vi "Process.vi"(0 "reference in":refnum<class "ACIR_EIS.lvclass">, 5 "error in":errorcluster) -> (14 "reference out":refnum<class "ACIR_EIS.lvclass">, 19 "error out":errorcluster)   [LabVIEW 2023, in "ACIR_EIS.lvclass"]
uses:
  ACIR_EIS.lvclass
  Types/EIS Mode.ctl
  Types/EIS Parameters.ctl
  Logger_class/Logger.lvclass
  <instrlib>/HPS-17000/HPS-17000.lvclass
  <vilib>/HPS-17000/nibatterycycler_grpc_Setpoint.ctl
  <vilib>/HPS-17000/Setpoint Stream Basic Config.ctl
  <vilib>/Utility/NIReport.llb/Report Type.ctl
  <instrlib>/HPS-17000/Internal/Set Energized Multi.vi
  <instrlib>/HPS-17000/Internal/Wait Until Energized Multi.vi
  <instrlib>/HPS-17000/Internal/Read Measurement Multi.vi
  <instrlib>/HPS-17000/Internal/Set Enabled Output Multi.vi
  <instrlib>/HPS-17000/Internal/Start Setpoint Stream Multi.vi
  <instrlib>/HPS-17000/Internal/Stream Setpoints Multi.vi
  <instrlib>/HPS-17000/Internal/Stop Setpoint Stream Multi.vi
  <instrlib>/HPS-17000/Internal/Write Setpoint Multi.vi
  <vilib>/printing/OpenHTMLReport.llb/Open HTML Report in Browser (Refnum).vi
  <vilib>/Utility/NIReport.llb/NI_report.lvclass
  ACIR_EIS.lvclass/ACIR_EIS.ctl
  <vilib>/Utility/SystemLogging/NI_SystemLogging.lvlib
  <vilib>/HPS-17000/NI_BC_client.lvlib
  <userlib>/_OpenG.lib/time/time.llb/openg_time.lvlib
  <vilib>/HPS-17000/Cycler.lvclass
  <vilib>/Utility/NIReport.llb/NI_ReportGenerationCore.lvlib
panel:
  out "Last Command":string
  out "error info":errorcluster
  in  "Save EIS Report":bool
  in  "EIS Tab Control":T1(tab)
  out "EIS Parameters":T3={"EIS Mode"=2, "EIS DC Potential"=650.0, "EIS Start Frequency"=1000.0, "EIS Stop Frequency"=500.0, "EIS Delta Frequency"=100.0, "EIS DC Current"=0.0, "AC Signal (mV/mA RMS)"=20.0, "Cycles at Frequency"=5.0, "EIS AC Step Delay"=1.0} {"EIS Mode" items=["Voltage (PEIS)"=1, "Current (GEIS)"=2]}
  out "EIS Profile":waveform(dbl)[](graph)
  out "Running Status Log":i32(listbox) caption="TEST SERVER LOG"
  out "EIS Step":dbl[][](graph)
  out "EIS Nyquist":cluster{dbl[], dbl[]}(graph)
  out "EIS Phase":cluster{dbl[], dbl[]}(graph)
  out "EIS Magnitude":cluster{dbl[], dbl[]}(graph)
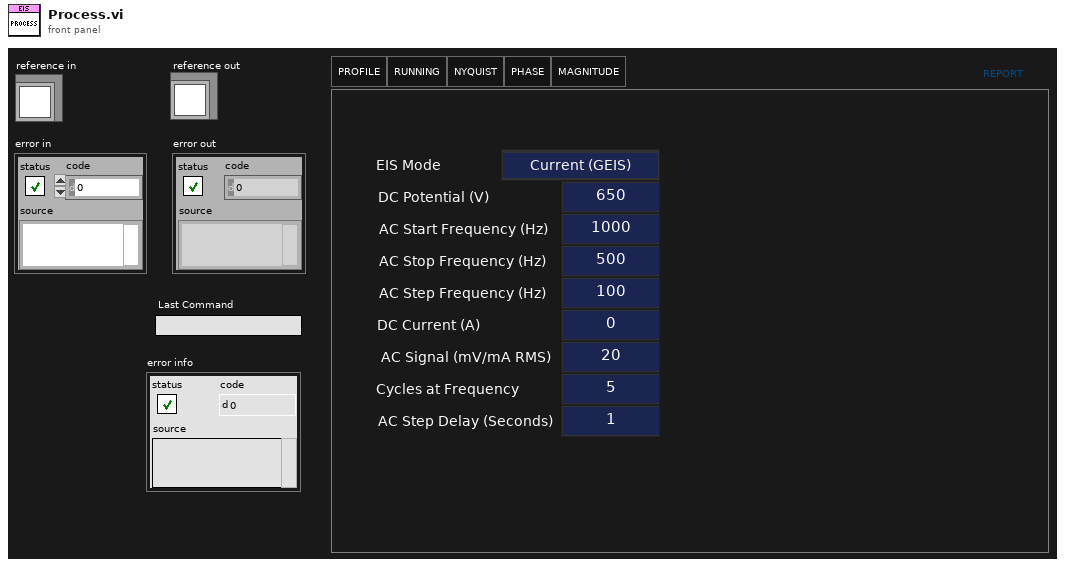
[diagram p1: front panel]
types:
  T1 = enum32{"PARAM", "PROFILE", "RUNNING", "NYQUIST", "PHASE", "MAGNITUDE"}
  T2 = typedef "EIS Mode.ctl" = u16
  T3 = cluster{"EIS Mode":T2, "EIS DC Potential":dbl, "EIS Start Frequency":dbl, "EIS Stop Frequency":dbl, "EIS Delta Frequency":dbl, "EIS DC Current":dbl, "AC Signal (mV/mA RMS)":dbl, "Cycles at Frequency":dbl, "EIS AC Step Delay":dbl}
  T4 = typedef "EIS Parameters.ctl" = cluster{"EIS Mode":T2, "EIS DC Potential":dbl, "EIS Start Frequency":dbl, "EIS Stop Frequency":dbl, "EIS Delta Frequency":dbl, "EIS DC Current":dbl, "AC Signal (mV/mA RMS)":dbl, "Cycles at Frequency":dbl, "EIS AC Step Delay":dbl}
  T5 = cluster{"Core":cluster{"Timeout":i32, "Events":cluster{"EventsToProcess":refnum<event-registration>}, "EventFromProcess":refnum<user-event>, "ProcessSyncQueue":refnum<queue>, "QueueFromProcess":refnum<queue>, "Command":string, "Data":variant}, "EIS Parameters":T4, "Profile Complete Event":refnum<user-event>, "EIS Profile State":enum16{"Idle", "Start", "Run", "Stop"}, "EIS TDMS Path":path, "Logger":refnum<class "Logger.lvclass">, "HPS17K Refs":refnum<class "HPS-17000.lvclass">[], "Voltage Profile":waveform(dbl)[], "Current Profile":waveform(dbl)[], "Next Step Timestamp":i64, "Profile Index":i64, "Frequencies":dbl[]}
  T6 = typedef "Cycler.lvclass/Setpoint Stream Basic Config.ctl" = cluster{"local address":string, "receiver port":u16}
  T7 = typedef "NI_BC_client.lvlib/nibatterycycler_grpc_Setpoint.ctl" = cluster{"voltage":sgl, "current":sgl, "min_power":sgl, "max_power":sgl, "resistance":sgl}
  T8 = enum8{"Enabled", "Disabled", "Disabled and Grayed Out"}
  T9 = typedef "NI_ReportGenerationCore.lvlib/Report Type.ctl" = enum16{"HTML", "Word", "Excel"}
  T10 = enum32{"Invalid", "Standard", "Closed", "Hidden", "Minimized", "Maximized"}
  T11 = cluster{"EventsToProcess":refnum<event-registration>}
  T12 = typedef "NI_BC_client.lvlib/MStream_grpc_CyclerMeasurement.ctl" = cluster{"measured_voltage":sgl, "measured_current":sgl, "setpoint_voltage":sgl, "setpoint_current":sgl, "timestamp":i64}
  T13 = typedef "ACIR_EIS.lvclass/ObjectAttributes.ctl" = cluster{"EIS Parameters":T4, "Logger":refnum<class "Logger.lvclass">, "HPS17K Refs":refnum<class "HPS-17000.lvclass">[]}
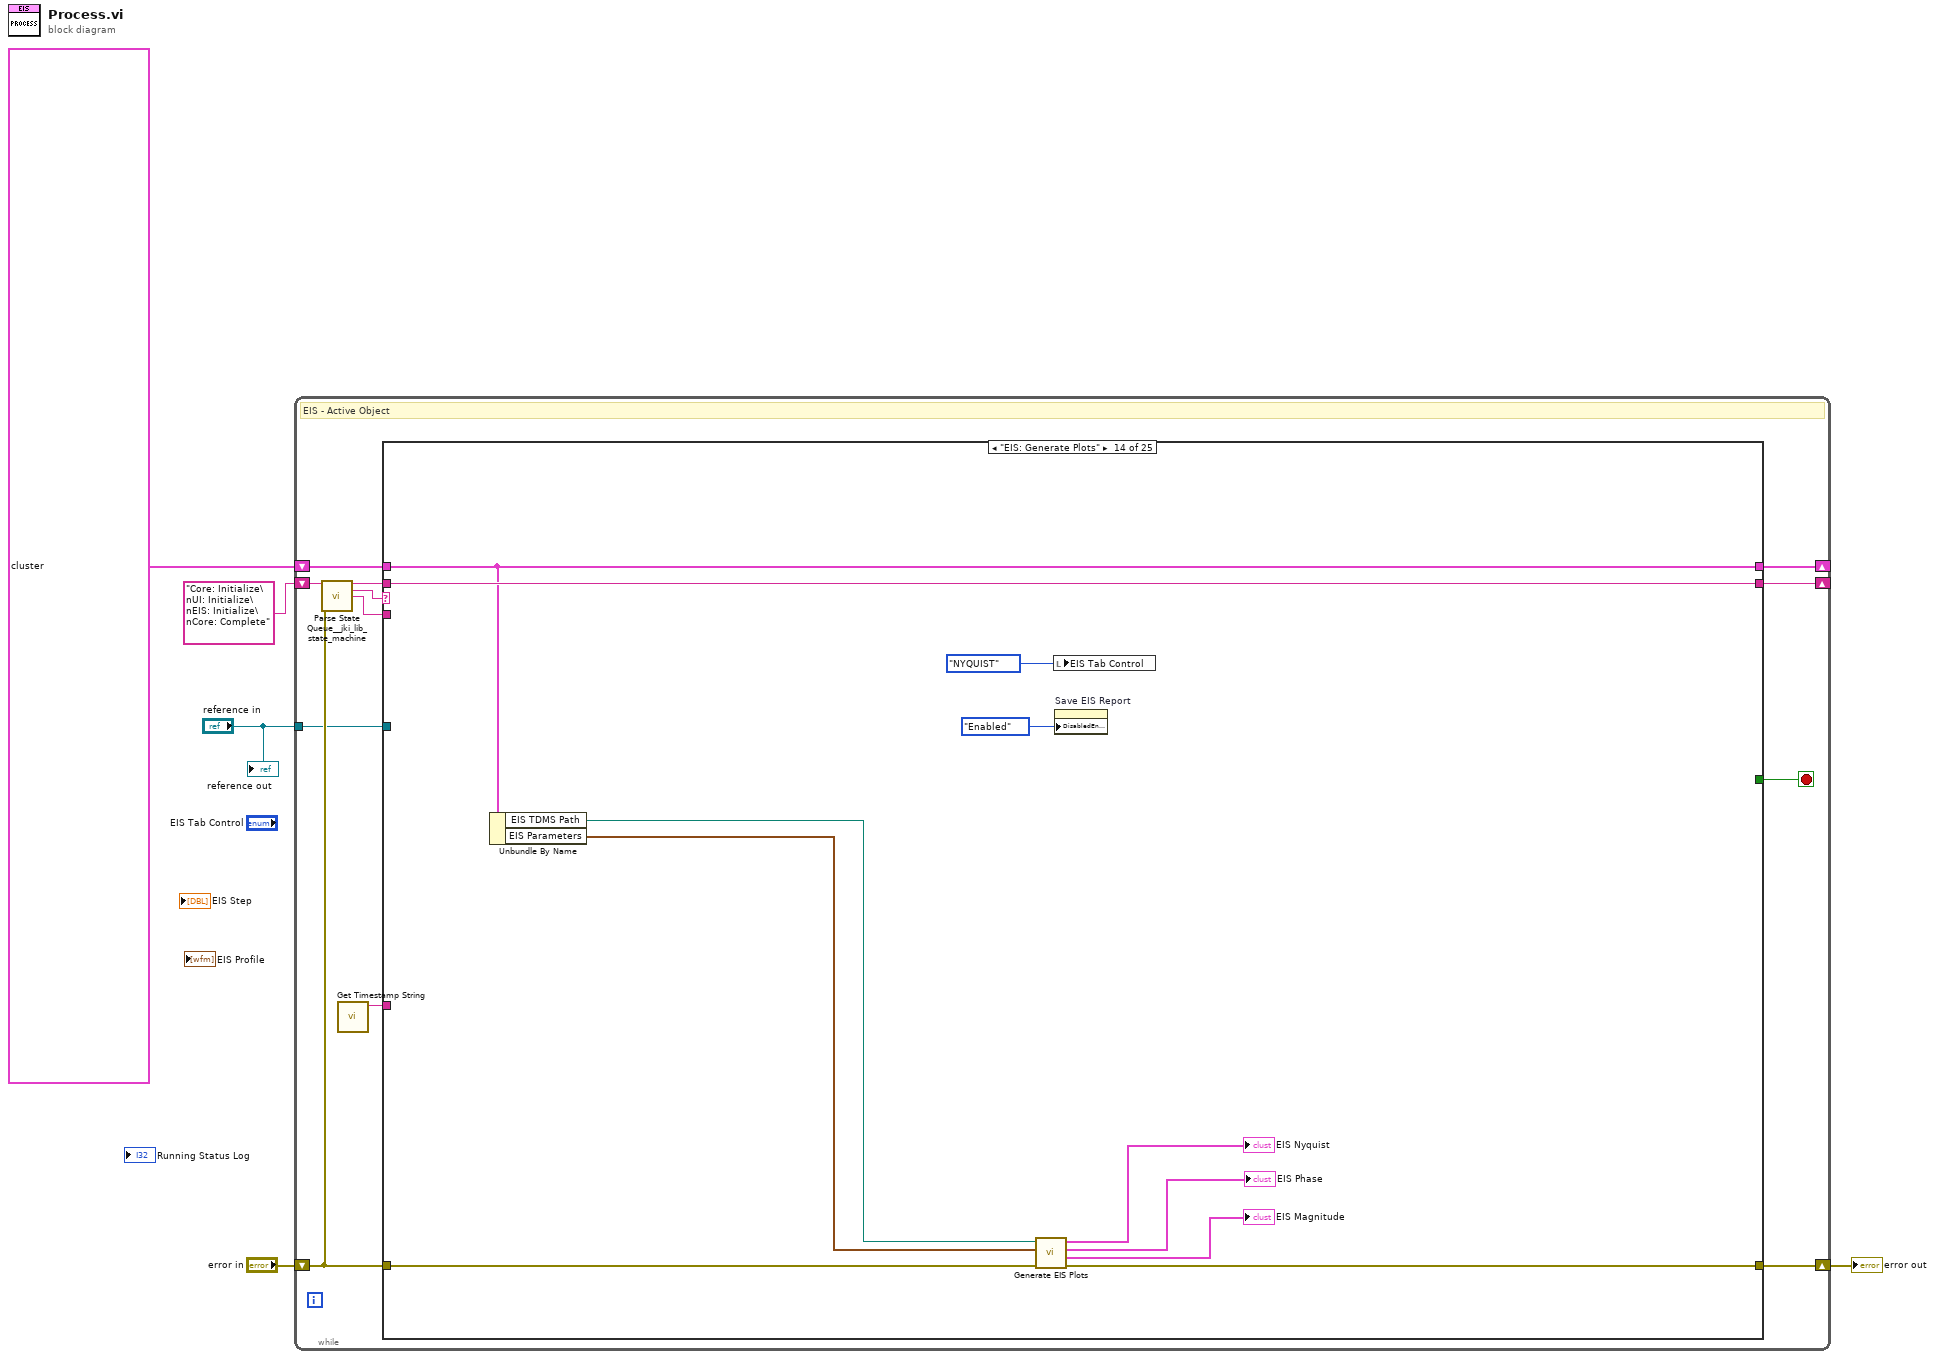
[diagram p0: block diagram]
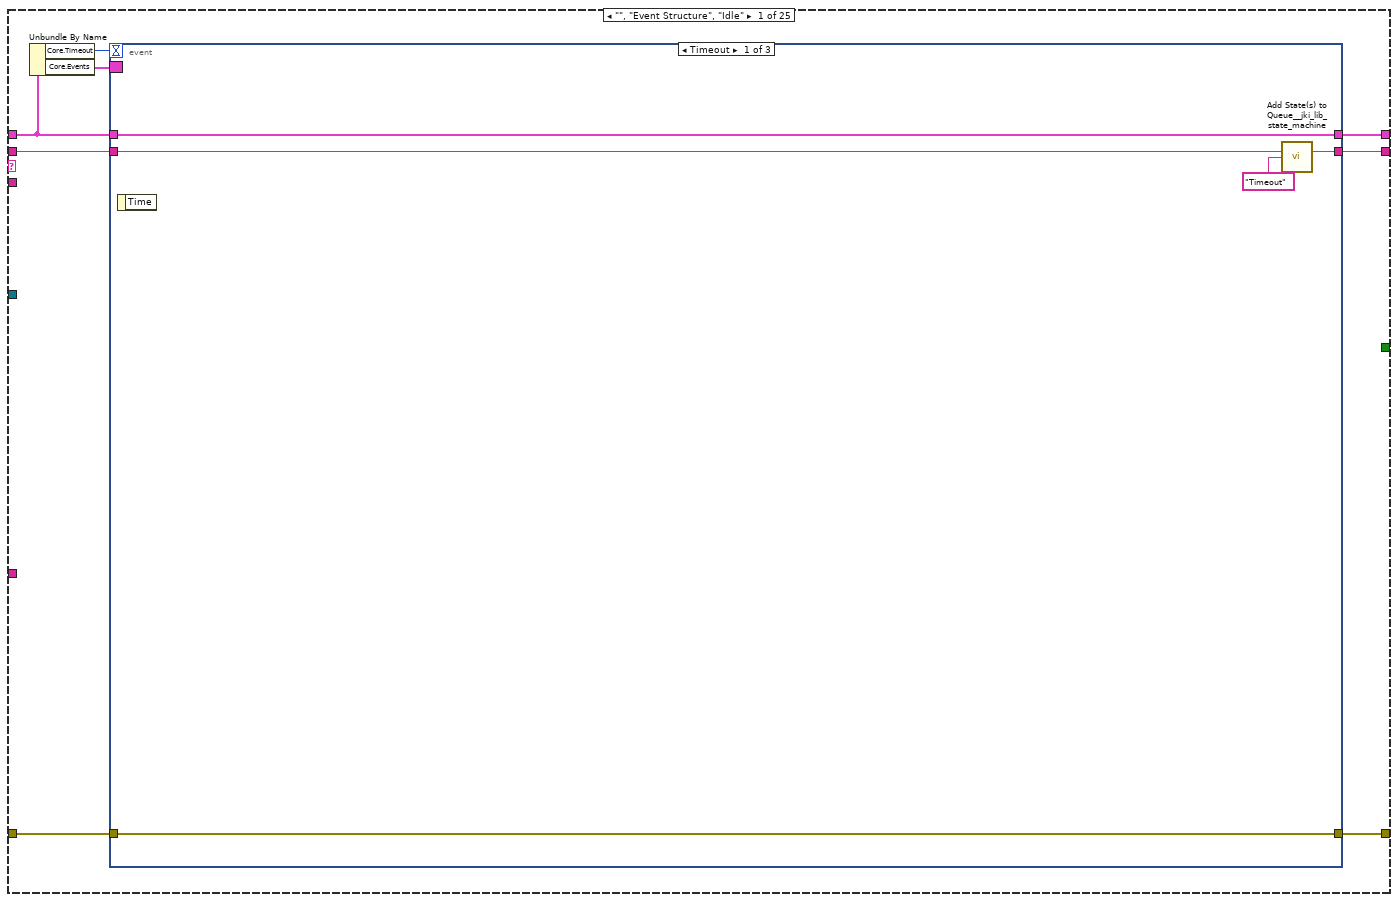
[diagram p2: hidden frame]
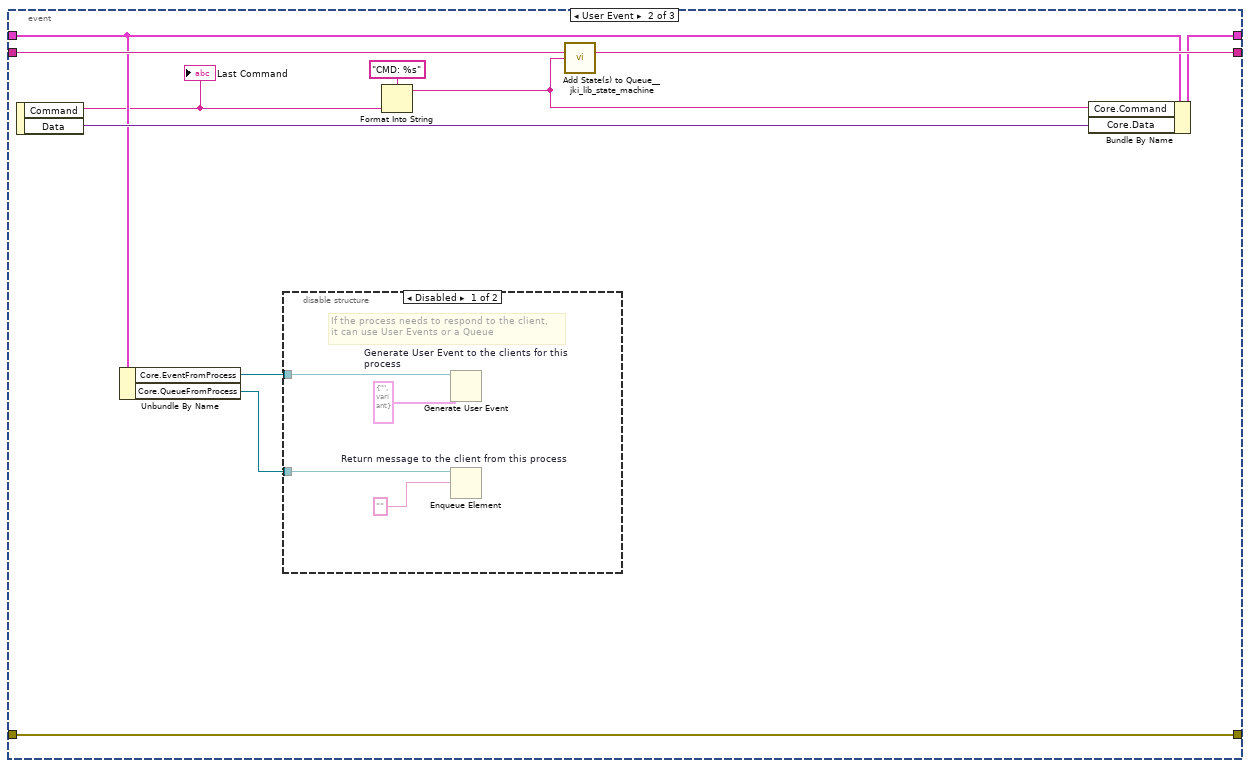
[diagram p3: hidden frame]
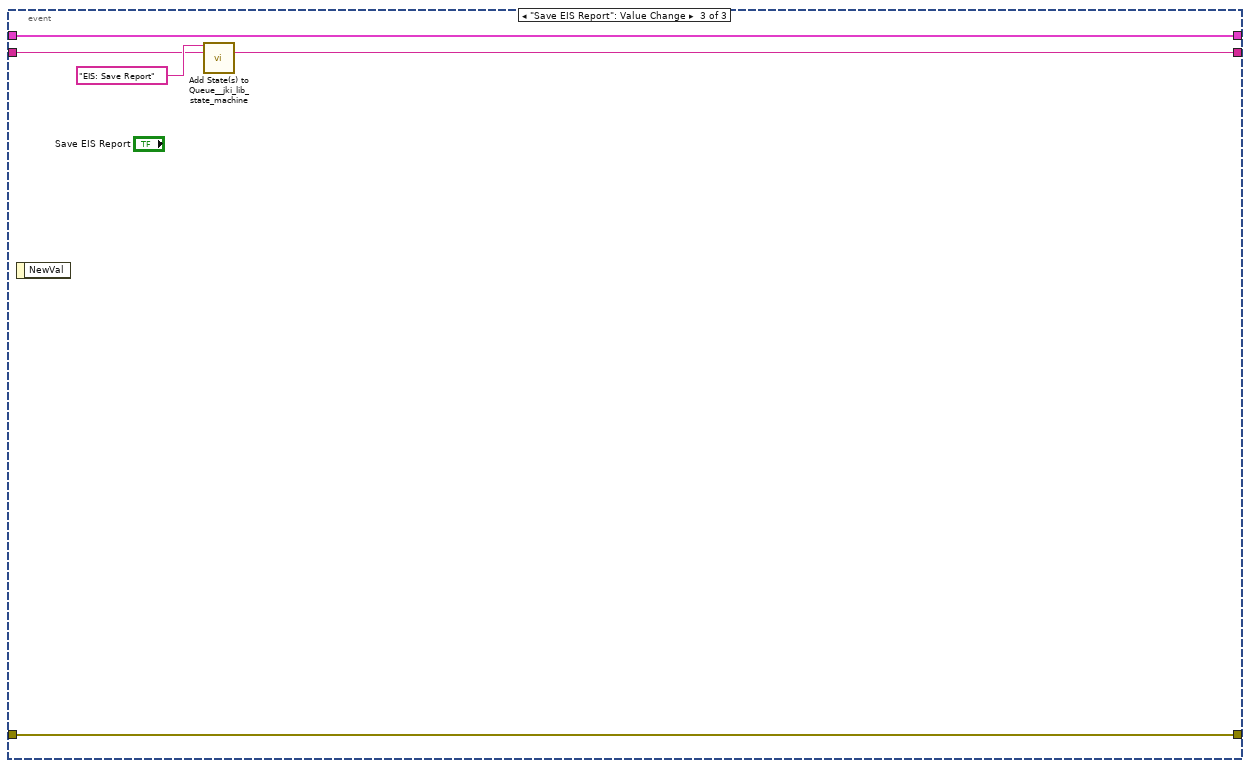
[diagram p5: hidden frame]
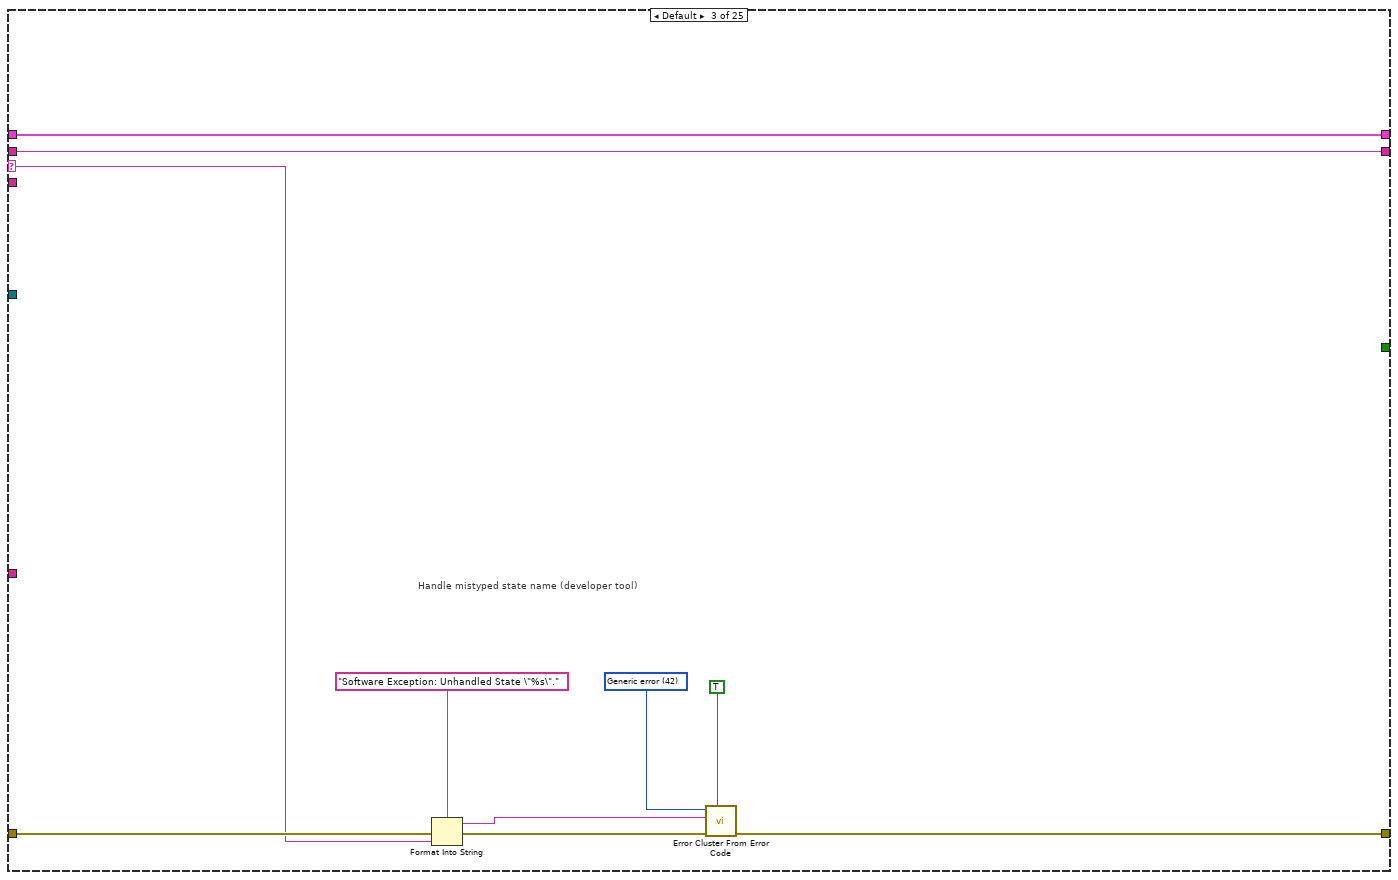
[diagram p7: hidden frame]
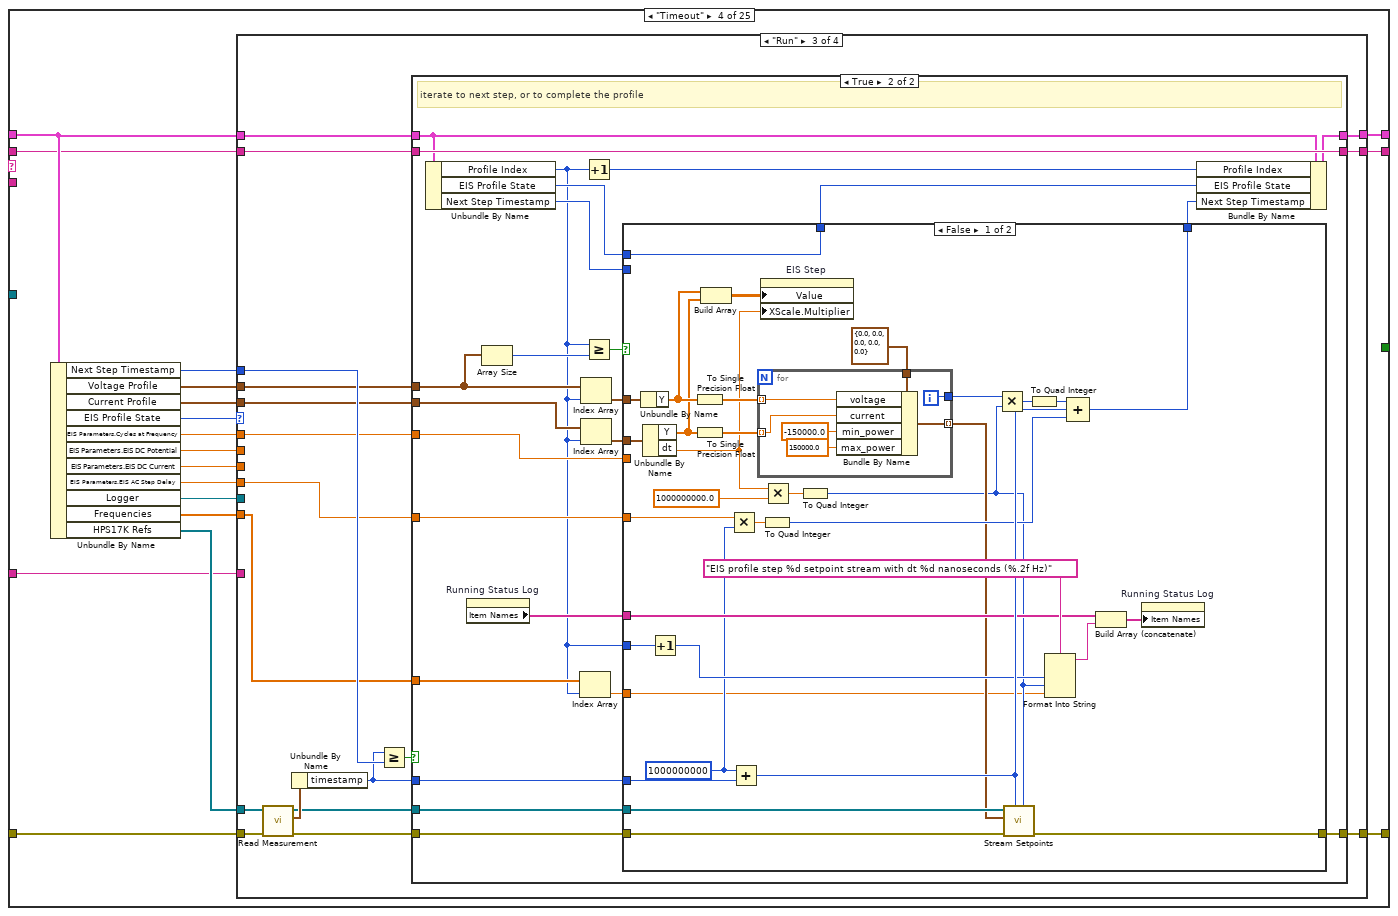
[diagram p8: hidden frame]
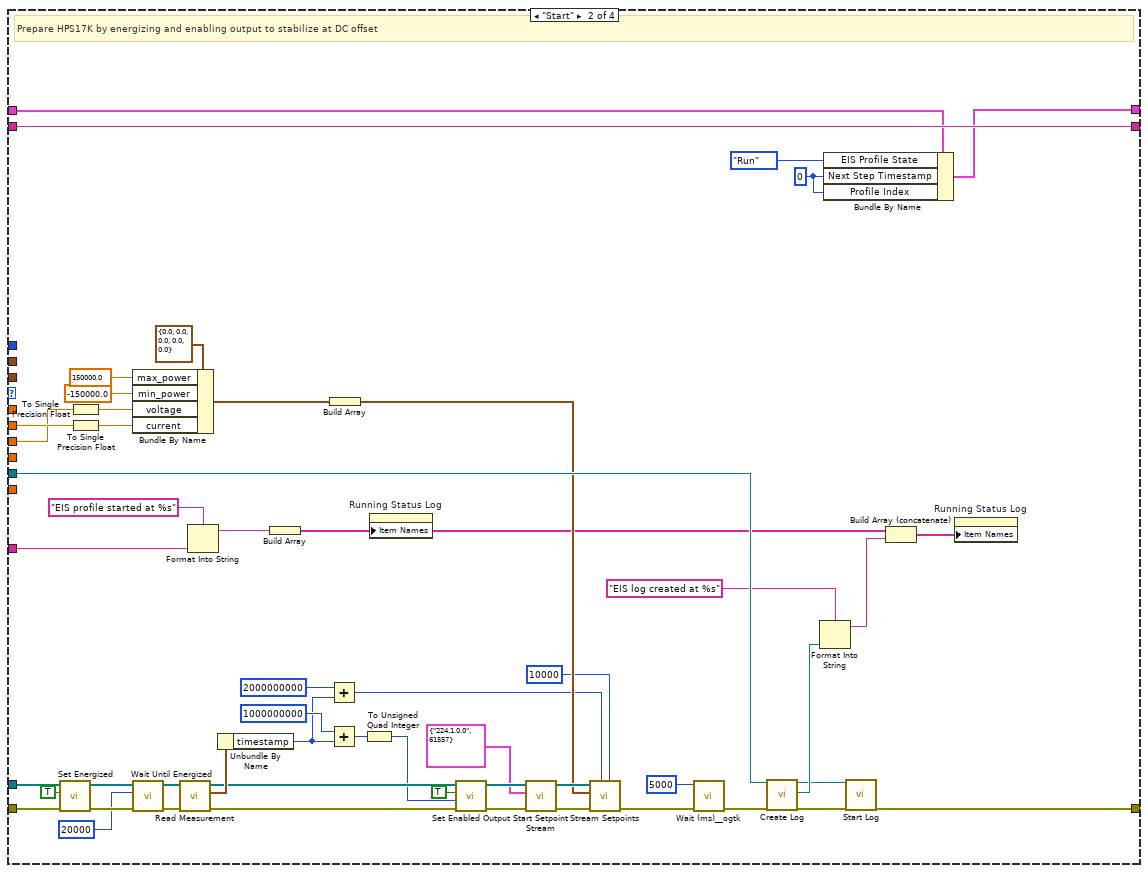
[diagram p10: hidden frame]
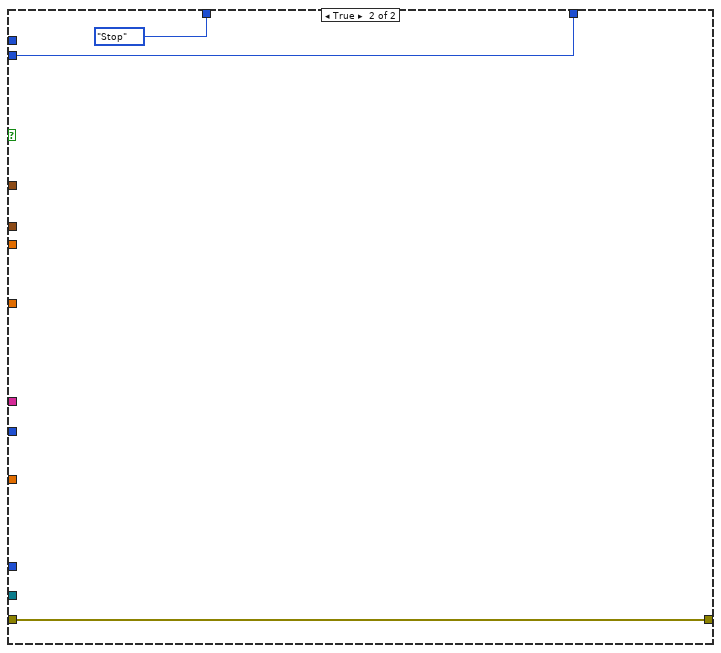
[diagram p12: hidden frame]
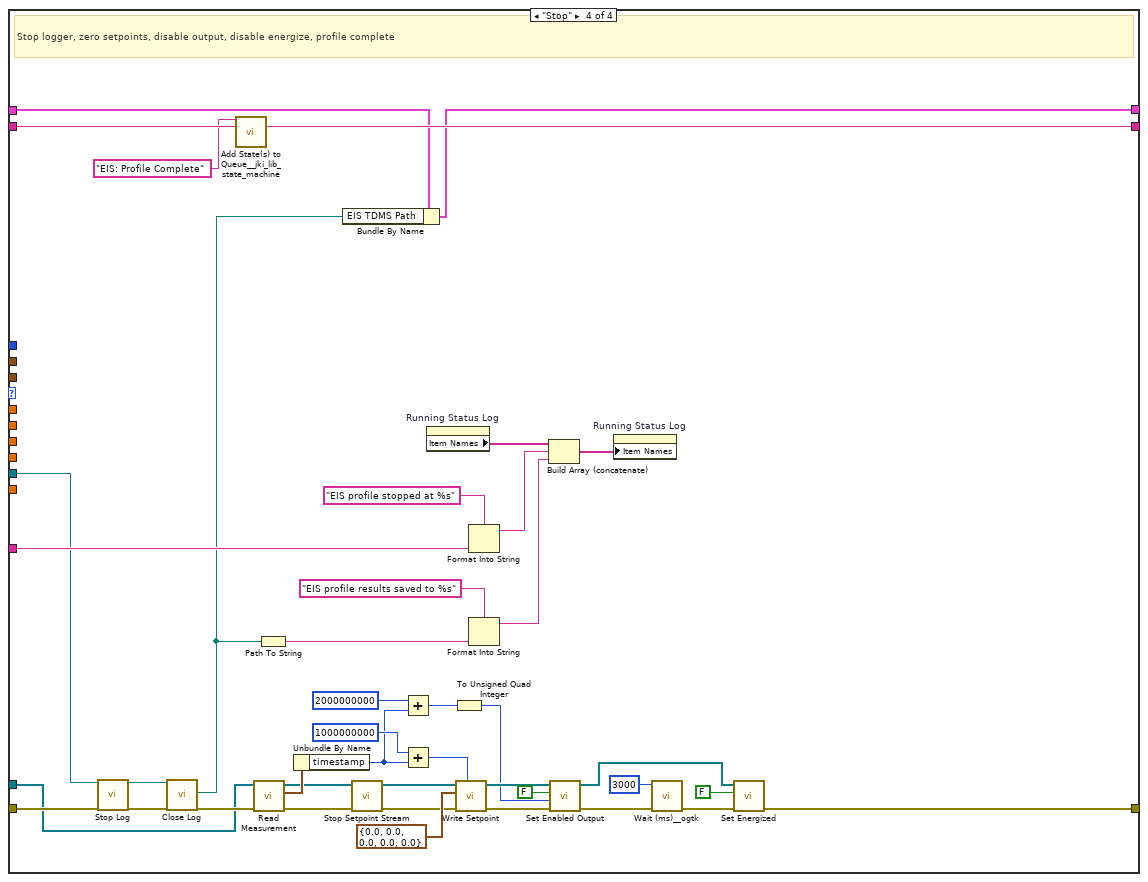
[diagram p13: hidden frame]
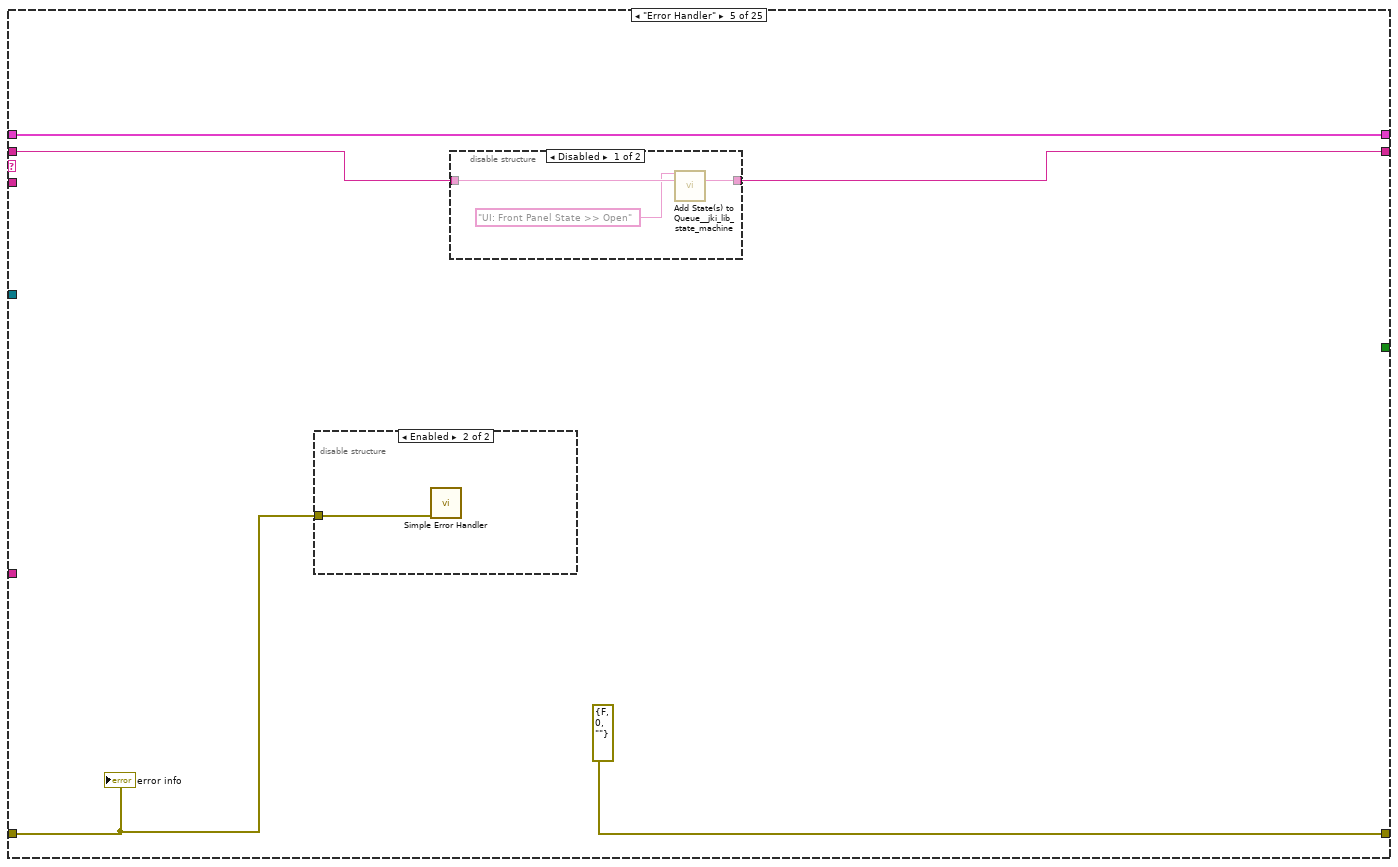
[diagram p14: hidden frame]
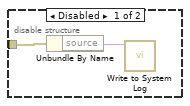
[diagram p16: hidden frame]
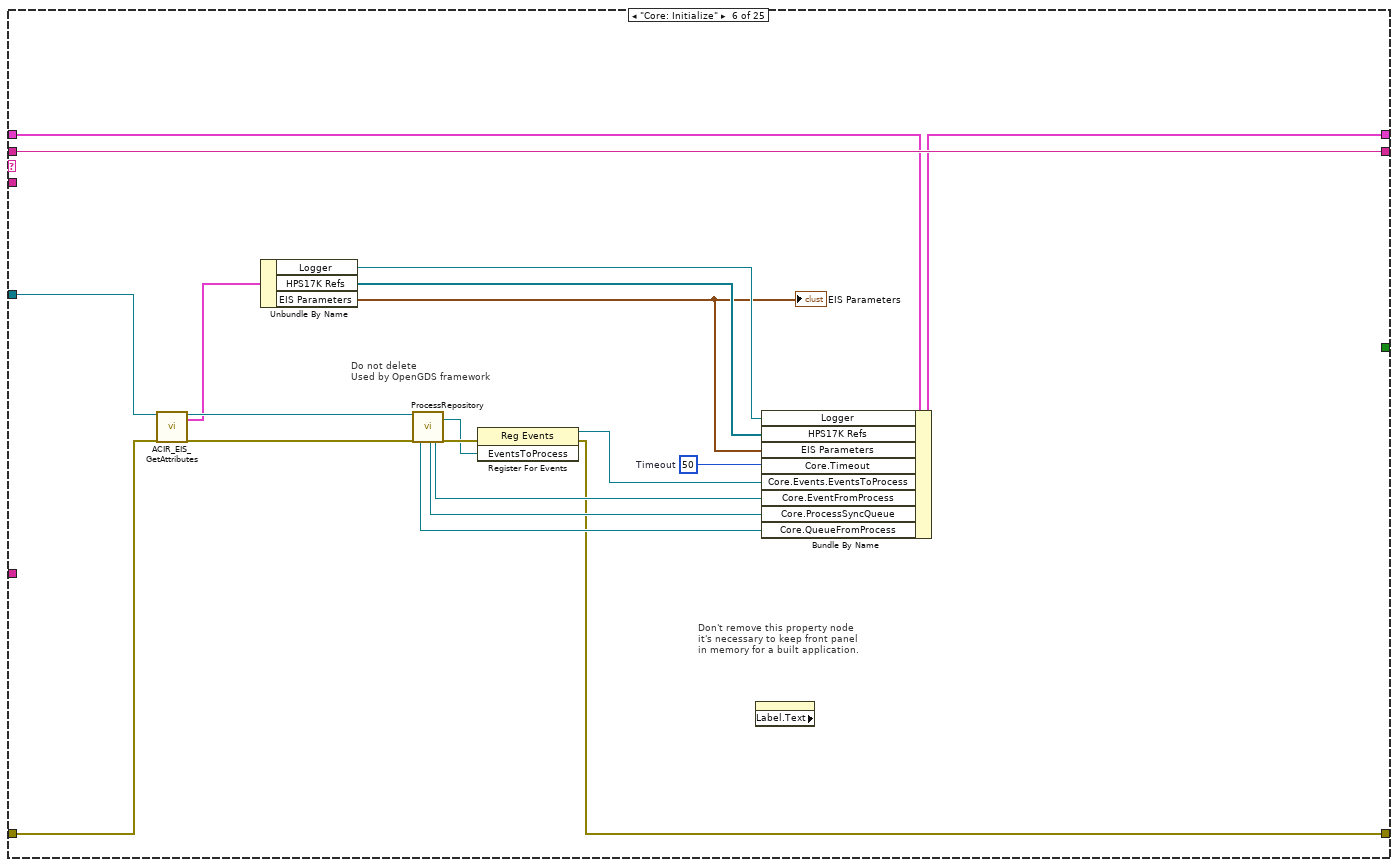
[diagram p17: hidden frame]
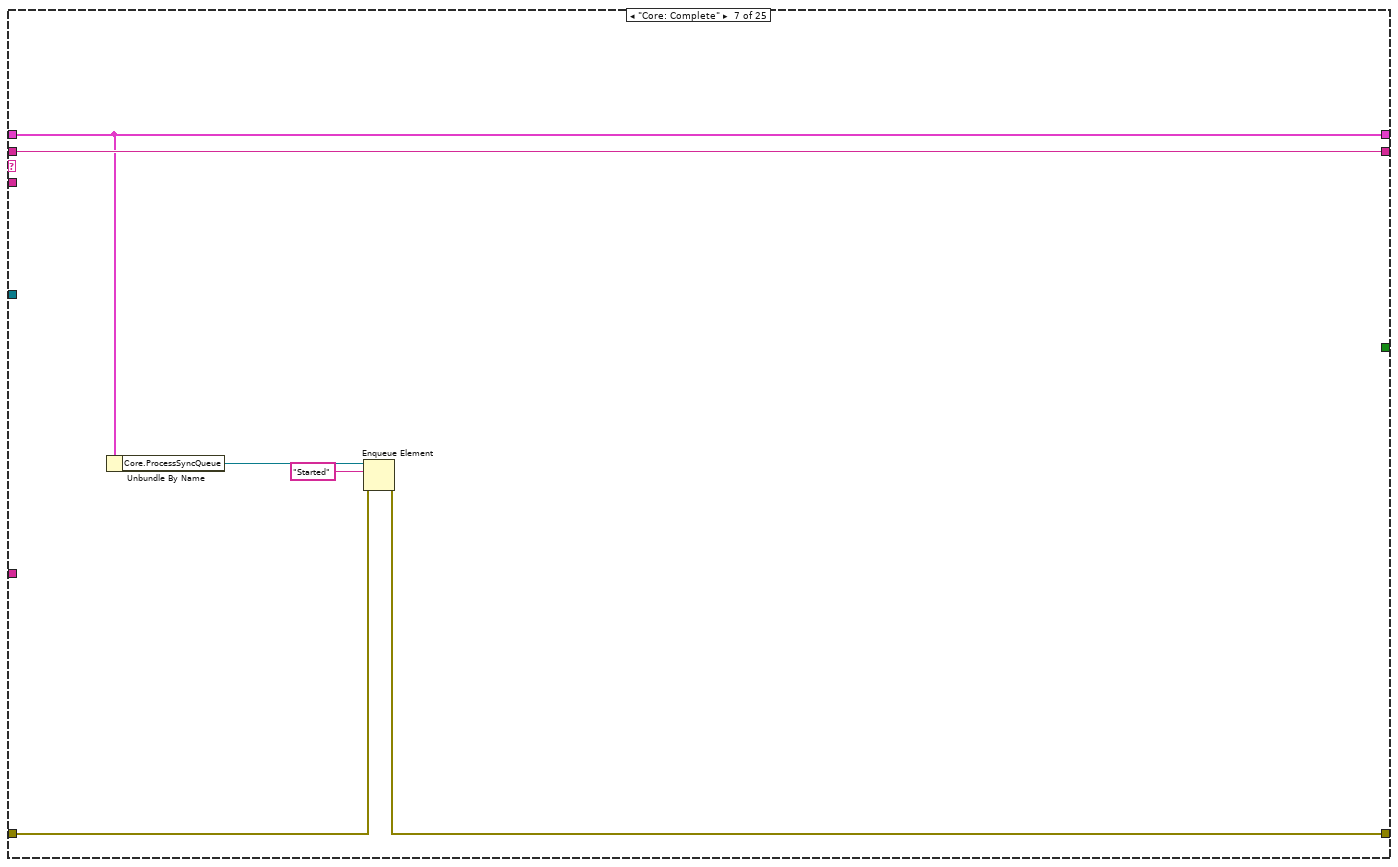
[diagram p18: hidden frame]
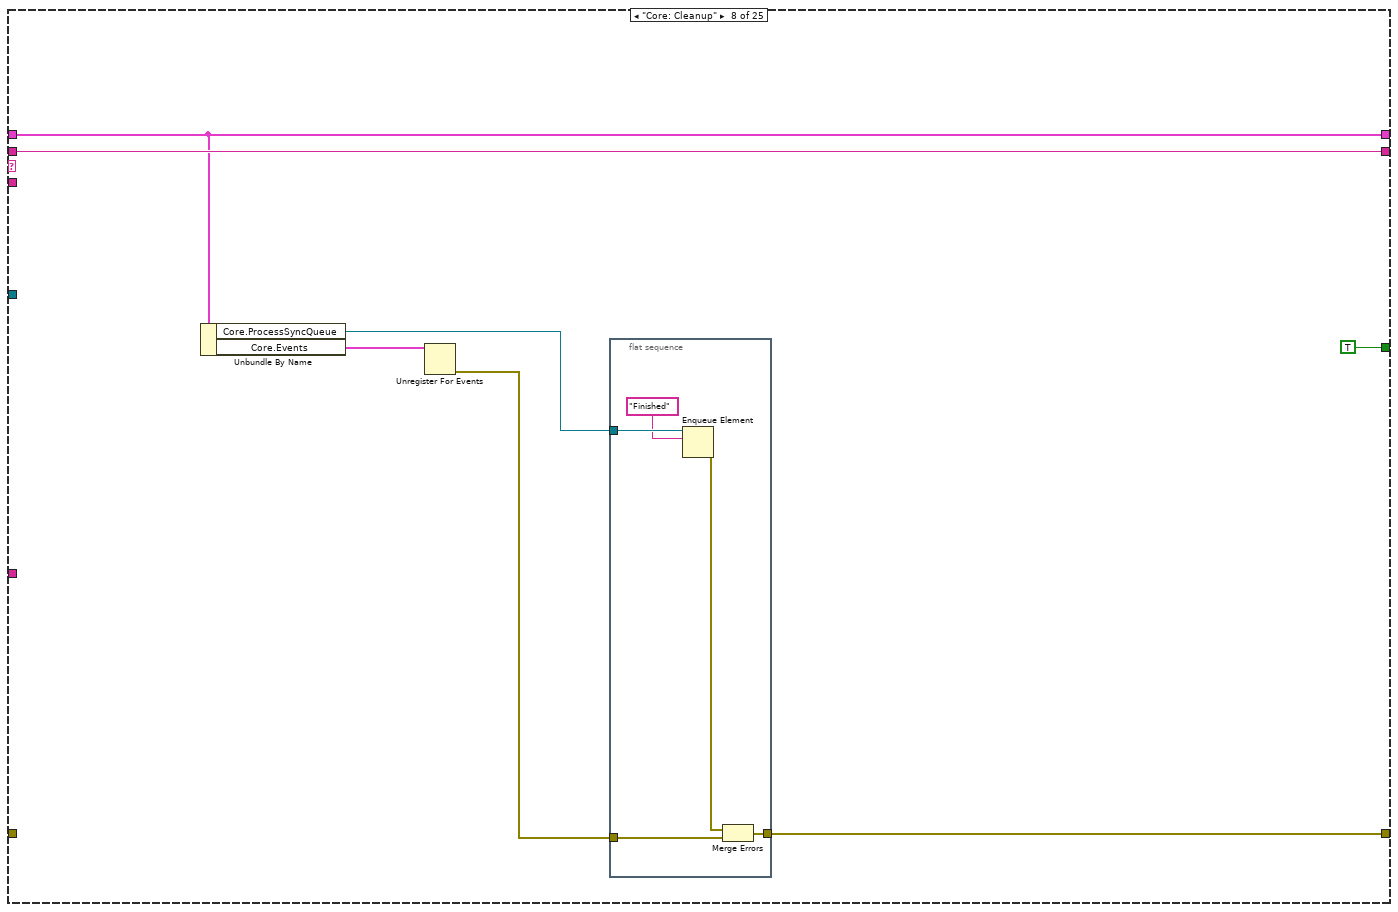
[diagram p19: hidden frame]
diagram:
  n1 = while {
    shift-right: [w16] -> w4
    shift-left: "error in" -> [w17]
    shift-right: [w9] -> _
    shift-left: "Core: Initialize\nUI: Initialize\nEIS: Initialize\nCore: Complete" ("States Out") -> [w12]
    shift-right: [w15] -> _
    shift-left: T5 {"Core"={"Timeout"=-1, "Events"={"EventsToProcess"=refnum}, "EventFromProcess"=refnum, "ProcessSyncQueue"=refnum, "QueueFromProcess"=refnum, "Command"="", "Data"=variant}, "EIS Parameters"={"EIS Mode"=2, "EIS DC Potential"=650.0, "EIS Start Frequency"=1000.0, "EIS Stop Frequency"=500.0, "EIS Delta Frequency"=100.0, "EIS DC Current"=0.0, "AC Signal (mV/mA RMS)"=20.0, "Cycles at Frequency"=1000.0, "EIS AC Step Delay"=1.0}, "Profile Complete Event"=refnum, "EIS Profile State"=enum."Idle", "EIS TDMS Path"=path "", "Logger"=refnum, "HPS17K Refs"=[], "Voltage Profile"=[], "Current Profile"=[], "Next Step Timestamp"=0, "Profile Index"=0, "Frequencies"=[]} ("LocalVariables") -> [w14]
    tunnel: "reference in" -> [w7]
    stop <- w8 stop-if-true
    # "EIS - Active Object"
    n2 = call <vilib>:"Parse State Queue__jki_lib_state_machine.vi"("State Queue"=w12, "Error In (no error)"=w17) -> ("Remaining States"=w11:string, "Current State"=w13:string, "Arguments"=w10:string)  [unwired: 11 in]
    n3 = call "Get Timestamp String.vi"() -> ("date/time string"=w6:string)  [unwired: 11 in]
    n4 = case shown="\"EIS: Generate Plots\"" w13 {
      selector: w13 -> [_ _ w54 _ _ _ _ _ _ _ _ _ _ _ _ _ _ _ _ _ _ _ _ _ _]
      tunnel: w17 -> [w19 w53 w56 w81 w269 w284 w300 _ w319 w330 w337 w342 w349 w361 w373 w432 w433 w461 _ w468 w471 w478 w486 w493 w498]
      tunnel: [w20 w53 w55 w80 errorcluster {"status"=FALSE, "code"=0, "source"=""} ("error constant") w289 w304 w307 w319 w329 w337 w342 w348 w359 w365 w432 w433 w461 w462 w468 w471 w478 w485 w493 w498] -> w16
      tunnel: [w25 w52 w63 w75 w272 w297 w301 w308 w318 w328 w334 w339 w346 w363 w375 w431 w435 w460 w463 w467 w470 w477 w483 w492 w497] -> w15
      tunnel: w14 -> [w21 w52 w63 w76 w272 w296 w301 w308 w318 w324 w335 w340 w347 w363 w375 w431 w435 w460 w463 w467 w470 w477 w484 w492 w497]
      tunnel: w11 -> [w23 w51 w62 w74 w271 w298 w303 w311 w317 w331 w336 w341 w353 w364 w374 w430 w436 w444 w465 w466 _ w476 w481 w491 w495]
      tunnel: w10 -> [_ _ _ _ _ _ _ _ _ _ _ _ _ _ _ _ w434 _ _ _ _ w473 _ _ _]
      tunnel: [w22 w51 w62 w73 w270 w298 w303 w311 w317 w331 w336 w341 w353 w364 w374 w430 w436 w444 w465 w466 "UI: Cleanup\nCore: Cleanup" ("State(s) at Back (\"\")") w475 w480 w490 w494] -> w9
      tunnel: [_ _ _ _ _ _ _ TRUE _ _ _ _ _ _ _ _ _ _ _ _ _ _ _ _ _] -> w8
      tunnel: w7 -> [_ _ _ _ _ w287 _ _ _ _ _ _ _ _ _ _ _ _ _ _ _ _ _ _ _]
      tunnel: w6 -> [_ _ _ w77 _ _ _ _ _ _ _ _ _ _ w367 _ _ _ _ _ _ _ _ _ _]
      frame "", "Event Structure", "Idle" {
        n5 = Unbundle By Name(w21) -> ("Core.Timeout"=w18:i32, "Core.Events"=w24:T11)
        n6 = event shown="[0] Timeout" {
          selector: w24 -> [_ _ _]
          dyn-events: _ -> [_ _ _]
          timeout: w18 -> [_ _ _]
          tunnel: w21 -> [w30 w34 w50]
          tunnel: [w30 w39 w50] -> w25
          tunnel: [w28 w41 w46] -> w22
          tunnel: w23 -> [w29 w40 w47]
          tunnel: [w26 w35 w49] -> w20
          tunnel: w19 -> [w26 w35 w49]
          event Timeout {
            n7 = event-data() -> ()  [unwired: 1 in, 1 out]
            n8 = call <vilib>:"Add State(s) to Queue__jki_lib_state_machine.vi"("State(s) in (\"\")"=w29, "State(s) at Back (\"\")"="Timeout" ("State(s) at Back (\"\")")) -> ("States Out"=w28:string)  [unwired: 13 in]
          }
          event User Event {
            n9 = event-data() -> ("Command"=w32:string, "Data"=w38:variant)  [unwired: 1 in]
            "Last Command" <- w32
            n10 = Unbundle By Name(w34) -> ("Core.EventFromProcess"=w37:refnum<user-event>, "Core.QueueFromProcess"=w36:refnum<queue>)
            n11 = disable-structure shown="Disabled" {
              disable-tunnel: w37 -> [w45 _]
              disable-tunnel: w36 -> [w44 _]
              frame Disabled {
                # "If the process needs to respond to the client,\nit can use User Events or a Queue"
                n12 = Generate User Event "Generate User Event to the clients for this process"(user event=w45, event data cluster=cluster{"Command":string, "Data":variant} {"Command"="", "Data"=variant} ("event data")) -> ()  [unwired: 2 in, 2 out]
                n13 = Enqueue Element "Return message to the client from this process"(queue=w44, element="") -> ()  [unwired: 2 in, 3 out]
              }
              frame Enabled {
              }
            }
            n14 = Format Into String(format string="CMD: %s", w32) -> (resulting string=w31:string)  [unwired: 2 in, 1 out]
            n15 = call <vilib>:"Add State(s) to Queue__jki_lib_state_machine.vi"("State(s) in (\"\")"=w40, "State(s) at Back (\"\")"=w31) -> ("States Out"=w41:string)  [unwired: 13 in]
            n16 = Bundle By Name(cluster=w34, "Core.Command"=w31, "Core.Data"=w38) -> (w39:T5)
          }
          event "Save EIS Report": Value Change {
            n17 = event-data() -> ()  [unwired: 1 in, 1 out]
            n18 = call <vilib>:"Add State(s) to Queue__jki_lib_state_machine.vi"("State(s) in Front (\"\")"="EIS: Save Report" ("State(s) in Front (\"\")"), "State(s) in (\"\")"=w47) -> ("States Out"=w46:string)  [unwired: 13 in]
          }
        }
      }
      frame "---------- Core ----------" {
      }
      frame Default {
        w60 = 42 items=["No error", "Argument error", "Memory is full", "Out of zone", "End of file", "File already open", "Generic file I/O error", "File not found", "File permission error", "Disk is full", "Duplicate path", "Too many files open", "System feature not enabled", "Resource file not found", "Cannot add resource", "Resource not found", "Image not found", "Image memory error", "Pen does not exist", "Config type invalid", "Config token not found", "Config parse error", "Config memory error", "Bad external code format", "Bad external code offset", "External code not present", "Null window", "Destroy window error", "Null menu", "Print aborted", "Bad print record", "Print driver error", "Windows error during printing", "Memory error during printing", "Print dialog error", "Generic print error", "Invalid device refnum", "Device not found", "Device parameter error", "Device unit error", "Cannot open device", "Device call aborted", "Generic error", "Cancelled by user", "Object ID too low", "Object ID too high", "Object not in heap", "Unknown heap", "Unknown object (invalid DefProc)", "Unknown object (DefProc not in table)", "Message out of range", "Invalid (null) method", "Unknown message", "Manager call not supported", "Bad address", "Network operation in progress", "Network operation timed out", "Connection is busy", "Network attribute not supported", "Network error", "Address in use", "System out of memory", "Connection aborted", "Connection refused", "Not connected", "Already connected", "Connection closed", "Initialization error (interapplication manager)", "Bad occurrence", "Wait on unbound occurrence handler", "Occurrence queue overflow", "Datalog type conflict", "Unused", "Unrecognized type (interapplication manager)", "Memory corrupt", "Failed to make temporary DLL", "Old CIN version", "Drag socket not found", "Failed to load drop-object", "Failed to register OLE object", "Failed to release OLE object", "Format specifier type mismatch", "Unknown format specifier", "Too few format specifiers", "Too many format specifiers", "Scan failed", "Newer CIN version", "Error converting to variant", "Runtime menu error", "Password tampered", "Variant attribute not found", "Incompatible variant data type", "Event data is not available", "Event Store is not present", "Occurrence is not found", "Event Queue is not created", "Event info is not available", "Refnum passed is NULL", "Error retrieving Class GUID", "Error retrieving CoClass GUID", "Error retrieving TypeLib GUID.", "Bad built application magic bytes.", "Specific driver is different from the specific driver associated with the Logical Name.", "There is no session opened to the class driver.", "Max Error", "MAX - Error with config objects", "MAX - Error loading configuration", "MAX - Group not supported"]
        # "Handle mistyped state name (developer tool)"
        n19 = Format Into String(format string="Software Exception: Unhandled State \"%s\"." ("message"), error in=w56, w54) -> (resulting string=w59:string, error out=w58:errorcluster)  [unwired: 1 in]
        n20 = call <vilib>:"Error Cluster From Error Code.vi"("show call chain? (False)"=TRUE, "error in (no error)"=w58, "error message (\"\")"=w59, "error code (0)"=w60) -> ("error out"=w55:errorcluster)  [unwired: 5 in]
      }
      frame "Timeout" {
        n21 = Unbundle By Name(w76) -> ("Next Step Timestamp"=w69:i64, "Voltage Profile"=w70:waveform(dbl)[], "Current Profile"=w71:waveform(dbl)[], "EIS Profile State"=w79:enum16{"Idle", "Start", "Run", "Stop"}, "EIS Parameters.Cycles at Frequency"=w65:dbl, "EIS Parameters.EIS DC Potential"=w66:dbl, "EIS Parameters.EIS DC Current"=w72:dbl, "EIS Parameters.EIS AC Step Delay"=w67:dbl, "Logger"=w68:refnum<class "Logger.lvclass">, "Frequencies"=w64:dbl[], "HPS17K Refs"=w78:refnum<class "HPS-17000.lvclass">[])
        n22 = case shown="\"Run\"" w79 {
          tunnel: w81 -> [w84 w100 w154 w259]
          tunnel: [w84 w115 w142 w233] -> w80
          tunnel: w78 -> [_ w99 w153 w251]
          tunnel: w68 -> [_ w126 _ w256]
          tunnel: w77 -> [_ w121 _ w263]
          tunnel: w76 -> [w83 w111 w150 w232]
          tunnel: [w83 w110 w149 w231] -> w75
          tunnel: w74 -> [w82 w114 w148 w262]
          tunnel: [w82 w114 w147 w260] -> w73
          tunnel: w72 -> [_ w108 _ _]
          tunnel: w66 -> [_ w107 _ _]
          tunnel: w71 -> [_ _ w143 _]
          tunnel: w70 -> [_ _ w144 _]
          tunnel: w69 -> [_ _ w152 _]
          tunnel: w67 -> [_ _ w140 _]
          tunnel: w65 -> [_ _ w139 _]
          tunnel: w64 -> [_ _ w138 _]
          frame "Idle", Default {
            # "do nothing"
          }
          frame "Start" {
            w106 = i64 0 ("Next Step Timestamp")
            # "Prepare HPS17K by energizing and enabling output to stabilize at DC offset"
            n23 = call-poly <instrlib>:"Set Energized.vi"("error in"=w100, "energize (T)"=TRUE, "cycler refs in"=w99) -> ("error out"=w131:errorcluster, "cycler refs out"=w130:refnum<class "HPS-17000.lvclass">[])  [unwired: 7 in]
            n24 = To Single Precision Float(number=w107) -> (single precision float=w136:sgl)
            n25 = To Single Precision Float(number=w108) -> (single precision float=w133:sgl)
            n26 = Bundle By Name(cluster=T7 {"voltage"=0.0, "current"=0.0, "min_power"=0.0, "max_power"=0.0, "resistance"=0.0} ("setpoint"), "max_power"=sgl 150000.0, "min_power"=sgl -150000.0 ("max_power"), "voltage"=w136, "current"=w133) -> (w93:T7)
            n27 = call-poly <instrlib>:"Wait Until Energized.vi"("error in"=w131, "timeout (ms)"=u32 20000, "cycler refs in"=w130) -> ("error out"=w98:errorcluster, "cycler refs out"=w97:refnum<class "HPS-17000.lvclass">[])  [unwired: 7 in]
            n28 = call-poly <instrlib>:"Read Measurement.vi"("error in"=w98, "cycler refs in"=w97) -> ("error out"=w96:errorcluster, "aggregated cycler measurements"=w132:T12, "cycler refs out"=w95:refnum<class "HPS-17000.lvclass">[])  [unwired: 7 in]
            n29 = Format Into String(format string="EIS profile started at %s", w121) -> (resulting string=w86:string)  [unwired: 2 in, 1 out]
            n30 = Unbundle By Name(w132) -> ("timestamp"=w101:i64)
            n31 = Build Array(w86) -> (w85:string[])
            n32 = Add(x=i64 2000000000, y=w101) -> (x+y=w90:i64)
            n33 = Add(x=i64 1000000000, y=w101) -> (x+y=w91:i64)
            n34 = Build Array(w93) -> (w92:T7[])
            n35 = To Unsigned Quad Integer(1:w91) -> (0:w89:u64)
            n36 = property on="Running Status Log" class="LstBox (strict)"("Item Names"=w85) -> ()  [unwired: 2 in, 2 out]
            n37 = call-poly <instrlib>:"Set Enabled Output.vi"("error in"=w96, "enabled timestamp"=w89, "enabled output"=TRUE, "cycler refs in"=w95) -> ("error out"=w105:errorcluster, "cycler refs out"=w104:refnum<class "HPS-17000.lvclass">[])  [unwired: 6 in]
            n38 = call-poly <instrlib>:"Start Setpoint Stream.vi"("error in"=w105, "setpoint stream config"=T6 {"local address"="224.1.0.0", "receiver port"=61557}, "cycler refs in"=w104) -> ("error out"=w102:errorcluster, "cycler refs out"=w94:refnum<class "HPS-17000.lvclass">[])  [unwired: 7 in]
            n39 = call-poly <instrlib>:"Stream Setpoints.vi"("dt"=i64 10000, "t0"=w90, "error in"=w102, "setpoints"=w92, "cycler refs in"=w94) -> ("error out"=w88:errorcluster)  [unwired: 5 in, 1 out]
            n40 = call <userlib>:"Wait (ms)__ogtk.vi"("error in (no error)"=w88, "milliseconds to wait"=u32 5000) -> ("error out"=w125:errorcluster)  [unwired: 8 in, 1 out]
            n41 = call "Create Log.vi"("reference in"=w126, "Error In"=w125) -> ("reference out"=w118:refnum<class "Logger.lvclass">, "created file"=w119:path, "Error Out"=w123:errorcluster)  [unwired: 15 in]
            n42 = Format Into String(format string="EIS log created at %s", w119) -> (resulting string=w117:string)  [unwired: 2 in, 1 out]
            n43 = Bundle By Name(cluster=w111, "EIS Profile State"=enum16{"Idle", "Start", "Run", "Stop"}."Run", "Next Step Timestamp"=w106, "Profile Index"=w106) -> (w110:T5)
            n44 = call "Start Log.vi"("reference in"=w118, "Error In"=w123) -> ("Error Out"=w115:errorcluster)  [unwired: 16 in, 1 out]
            n45 = Build Array (concatenate)(w85, w117) -> (w116:string[])
            n46 = property on="Running Status Log" class="LstBox (strict)"("Item Names"=w116) -> ()  [unwired: 2 in, 2 out]
          }
          frame "Run" {
            n47 = call-poly <instrlib>:"Read Measurement.vi"("error in"=w154, "cycler refs in"=w153) -> ("error out"=w146:errorcluster, "aggregated cycler measurements"=w155:T12, "cycler refs out"=w141:refnum<class "HPS-17000.lvclass">[])  [unwired: 7 in]
            n48 = Unbundle By Name(w155) -> ("timestamp"=w145:i64)
            n49 = Greater Or Equal?(x=w145, y=w152) -> (x >= y?=w151:bool)
            n50 = case shown="True" w151 {
              tunnel: w150 -> [w158 w181]
              tunnel: [w158 w179] -> w149
              tunnel: w148 -> [w157 w182]
              tunnel: [w157 w182] -> w147
              tunnel: w146 -> [w156 w174]
              tunnel: w145 -> [_ w167]
              tunnel: w144 -> [_ w172]
              tunnel: w143 -> [_ w171]
              tunnel: [w156 w173] -> w142
              tunnel: w141 -> [_ w168]
              tunnel: w140 -> [_ w166]
              tunnel: w139 -> [_ w162]
              tunnel: w138 -> [_ w161]
              frame False {
                # "wait until current step is completed, do nothing"
              }
              frame True {
                # "iterate to next step, or to complete the profile"
                n51 = Unbundle By Name(w181) -> ("Profile Index"=w160:i64, "EIS Profile State"=w175:enum16{"Idle", "Start", "Run", "Stop"}, "Next Step Timestamp"=w164:i64)
                n52 = property on="Running Status Log" class="LstBox (strict)"() -> ("Item Names"=w163:string[])  [unwired: 2 in, 2 out]
                n53 = Array Size(array=w172) -> (size(s)=w180:i32)
                n54 = Index Array(array=w161, index=w160) -> (element=w159:dbl)
                n55 = Index Array(array=w172, index=w160) -> (element=w170:waveform(dbl))
                n56 = Index Array(array=w171, index=w160) -> (element=w169:waveform(dbl))
                n57 = Increment(x=w160) -> (x+1=w178:i64)
                n58 = Greater Or Equal?(x=w160, y=w180) -> (x >= y?=w177:bool)
                n59 = case shown="False" w177 {
                  tunnel: [w216 enum16{"Idle", "Start", "Run", "Stop"}."Stop" ("EIS Profile State")] -> w176
                  tunnel: w175 -> [w216 _]
                  tunnel: w174 -> [w213 w225]
                  tunnel: [w212 w225] -> w173
                  tunnel: w170 -> [w215 _]
                  tunnel: w169 -> [w214 _]
                  tunnel: w168 -> [w211 _]
                  tunnel: w167 -> [w210 _]
                  tunnel: w166 -> [w206 _]
                  tunnel: [w200 w224] -> w165
                  tunnel: w164 -> [_ w224]
                  tunnel: w163 -> [w196 _]
                  tunnel: w160 -> [w195 _]
                  tunnel: w162 -> [_ _]
                  tunnel: w159 -> [w183 _]
                  frame False {
                    w192 = i64 1000000000 ("x")
                    n60 = Unbundle By Name(w215) -> ("Y"=w191:dbl[])
                    n61 = Unbundle By Name(w214) -> ("Y"=w190:dbl[], "dt"=w185:dbl)
                    n62 = Increment(x=w195) -> (x+1=w194:i64)
                    n63 = To Single Precision Float(number=w191) -> (single precision float=w208:sgl[])
                    n64 = To Single Precision Float(number=w190) -> (single precision float=w207:sgl[])
                    n65 = Build Array(w191, w190) -> (w187:dbl[][])
                    n66 = Multiply(x=w206, y=w192) -> (x*y=w205:dbl)
                    n67 = Add(x=w192, y=w210) -> (x+y=w201:i64)
                    n68 = for {
                      tunnel: w208 -> [w222] mode=indexing
                      tunnel: T7 {"voltage"=0.0, "current"=0.0, "min_power"=0.0, "max_power"=0.0, "resistance"=0.0} ("nibatterycycler_grpc_Setpoint") -> [w223]
                      tunnel: w207 -> [w221] mode=indexing
                      tunnel: [w218] -> w186 mode=indexing
                      tunnel: [w217] -> w204
                      i -> [w217]
                      n69 = Bundle By Name(cluster=w223, "voltage"=w222, "current"=w221, "min_power"=sgl -150000.0, "max_power"=sgl 150000.0) -> (w218:T7)
                    }
                    n70 = property on="EIS Step" class="WFGraph (strict)"("Value"=w187, "XScale.Multiplier"=w185) -> ()  [unwired: 2 in, 2 out]
                    n71 = To Quad Integer(1:w205) -> (0:w193:i64)
                    n72 = Multiply(x=w185, y=1000000000.0) -> (x*y=w188:dbl)
                    n73 = To Quad Integer(1:w188) -> (0:w184:i64)
                    n74 = Multiply(x=w204, y=w184) -> (x*y=w203:i64)
                    n75 = call-poly <instrlib>:"Stream Setpoints.vi"("dt"=w184, "t0"=w201, "error in"=w213, "setpoints"=w186, "cycler refs in"=w211) -> ("error out"=w212:errorcluster)  [unwired: 5 in, 1 out]
                    n76 = To Quad Integer(1:w203) -> (0:w202:i64)
                    n77 = Format Into String(format string="EIS profile step %d setpoint stream with dt %d nanoseconds (%.2f Hz)", w194, w184, w183) -> (resulting string=w199:string)  [unwired: 2 in, 1 out]
                    n78 = Compound Arithmetic op=ADD(w202, w201, w193) -> (w200:i64)
                    n79 = Build Array (concatenate)(w196, w199) -> (w198:string[])
                    n80 = property on="Running Status Log" class="LstBox (strict)"("Item Names"=w198) -> ()  [unwired: 2 in, 2 out]
                  }
                  frame True {
                  }
                }
                n81 = Bundle By Name(cluster=w181, "Profile Index"=w178, "EIS Profile State"=w176, "Next Step Timestamp"=w165) -> (w179:T5)
              }
            }
          }
          frame "Stop" {
            # "Stop logger, zero setpoints, disable output, disable energize, profile complete"
            n82 = call "Stop Log.vi"("reference in"=w256, "Error In"=w259) -> ("reference out"=w257:refnum<class "Logger.lvclass">, "Error Out"=w258:errorcluster)  [unwired: 16 in]
            n83 = call "Close Log.vi"("reference in"=w257, "Error In"=w258) -> ("log file path"=w227:path, "Error Out"=w252:errorcluster)  [unwired: 15 in, 1 out]
            n84 = call <vilib>:"Add State(s) to Queue__jki_lib_state_machine.vi"("State(s) in Front (\"\")"="EIS: Profile Complete" ("State(s) in Front (\"\")"), "State(s) in (\"\")"=w262) -> ("States Out"=w260:string)  [unwired: 13 in]
            n85 = call-poly <instrlib>:"Read Measurement.vi"("error in"=w252, "cycler refs in"=w251) -> ("error out"=w237:errorcluster, "aggregated cycler measurements"=w255:T12, "cycler refs out"=w236:refnum<class "HPS-17000.lvclass">[])  [unwired: 7 in]
            n86 = Path To String(path=w227) -> (string=w229:string)
            n87 = Unbundle By Name(w255) -> ("timestamp"=w246:i64)
            n88 = Bundle By Name(cluster=w232, "EIS TDMS Path"=w227) -> (w231:T5)
            n89 = call-poly <instrlib>:"Stop Setpoint Stream.vi"("error in"=w237, "cycler refs in"=w236) -> ("error out"=w235:errorcluster, "cycler refs out"=w234:refnum<class "HPS-17000.lvclass">[])  [unwired: 8 in]
            n90 = Add(x=i64 2000000000, y=w246) -> (x+y=w247:i64)
            n91 = Add(x=i64 1000000000, y=w246) -> (x+y=w254:i64)
            n92 = property on="Running Status Log" class="LstBox (strict)"() -> ("Item Names"=w267:string[])  [unwired: 2 in, 2 out]
            n93 = To Unsigned Quad Integer(1:w247) -> (0:w243:u64)
            n94 = call-poly <instrlib>:"Write Setpoint.vi"("timestamp"=w254, "error in"=w235, "setpoint"=T7 {"voltage"=0.0, "current"=0.0, "min_power"=0.0, "max_power"=0.0, "resistance"=0.0}, "cycler refs in"=w234) -> ("error out"=w245:errorcluster, "cycler refs out"=w244:refnum<class "HPS-17000.lvclass">[])  [unwired: 6 in]
            n95 = Format Into String(format string="EIS profile stopped at %s", w263) -> (resulting string=w266:string)  [unwired: 2 in, 1 out]
            n96 = Format Into String(format string="EIS profile results saved to %s", w229) -> (resulting string=w228:string)  [unwired: 2 in, 1 out]
            n97 = Build Array (concatenate)(w267, w266, w228) -> (w265:string[])
            n98 = call-poly <instrlib>:"Set Enabled Output.vi"("error in"=w245, "enabled timestamp"=w243, "enabled output"=FALSE, "cycler refs in"=w244) -> ("error out"=w241:errorcluster, "cycler refs out"=w239:refnum<class "HPS-17000.lvclass">[])  [unwired: 6 in]
            n99 = property on="Running Status Log" class="LstBox (strict)"("Item Names"=w265) -> ()  [unwired: 2 in, 2 out]
            n100 = call <userlib>:"Wait (ms)__ogtk.vi"("error in (no error)"=w241, "milliseconds to wait"=u32 3000) -> ("error out"=w240:errorcluster)  [unwired: 8 in, 1 out]
            n101 = call-poly <instrlib>:"Set Energized.vi"("error in"=w240, "energize (T)"=FALSE, "cycler refs in"=w239) -> ("error out"=w233:errorcluster)  [unwired: 7 in, 1 out]
          }
        }
      }
      frame "Error Handler" {
        n102 = disable-structure shown="Enabled" {
          disable-tunnel: w269 -> [w278 w279]
          frame Disabled {
            n103 = Unbundle By Name(w278) -> ("source"=w277:string)
            n104 = call <vilib>:"Write to System Log.vi"("message"=w277) -> ()  [unwired: 10 in, 1 out]
          }
          frame Enabled {
            n105 = call <vilib>:"Simple Error Handler.vi"("error in (no error)"=w279) -> ()  [unwired: 4 in, 5 out]
          }
        }
        n106 = disable-structure shown="Disabled" {
          disable-tunnel: w271 -> [w275 w276]
          disable-tunnel: [w274 w276] -> w270
          frame Disabled {
            n107 = call <vilib>:"Add State(s) to Queue__jki_lib_state_machine.vi"("State(s) in Front (\"\")"="UI: Front Panel State >> Open" ("State(s) at Back (\"\")"), "State(s) in (\"\")"=w275) -> ("States Out"=w274:string)  [unwired: 13 in]
          }
          frame Enabled {
          }
        }
        "error info" <- w269
      }
      frame "Core: Initialize" {
        w288 = 50  # Timeout
        # "Do not delete\nUsed by OpenGDS framework"
        # "Don't remove this property node\nit's necessary to keep front panel\nin memory for a built application."
        # "Template created by VI Technologies"
        n108 = call "ACIR_EIS_GetAttributes.vi"("reference in"=w287, "Error In"=w284) -> ("reference out"=w286:refnum<class "ACIR_EIS.lvclass">, "Data"=w283:T13, "Error Out"=w285:errorcluster)  [unwired: 14 in, 1 out]
        n109 = Unbundle By Name(w283) -> ("Logger"=w281:refnum<class "Logger.lvclass">, "HPS17K Refs"=w282:refnum<class "HPS-17000.lvclass">[], "EIS Parameters"=w280:T4)
        "EIS Parameters" <- w280
        n110 = call "ProcessRepository.vi"("reference in"=w286, "Error In"=w285) -> ("QueueFromProcess"=w291:refnum<queue>, "ProcessSyncQueue"=w290:refnum<queue>, "EventFromProcess"=w292:refnum<user-event>, "EventsToProcess"=w294:refnum<user-event>, "Error Out"=w295:errorcluster)  [unwired: 10 in, 3 out]
        n111 = register-events(error in=w295, w294) -> (reference out=w293:refnum<event-registration>, error out=w289:errorcluster)  [unwired: 1 in]
        n112 = property on="reference in" class="LVClassControl (strict)" props=["Label", "Text"]() -> ()  [unwired: 2 in, 3 out]
        n113 = Bundle By Name(cluster=w296, "Logger"=w281, "HPS17K Refs"=w282, "EIS Parameters"=w280, "Core.Timeout"=w288, "Core.Events.EventsToProcess"=w293, "Core.EventFromProcess"=w292, "Core.ProcessSyncQueue"=w290, "Core.QueueFromProcess"=w291) -> (w297:T5)
      }
      frame "Core: Complete" {
        # "Template created by VI Technologies"
        n114 = Unbundle By Name(w301) -> ("Core.ProcessSyncQueue"=w299:refnum<queue>)
        n115 = Enqueue Element(queue=w299, element="Started", error in (no error)=w300) -> (error out=w304:errorcluster)  [unwired: 1 in, 2 out]
      }
      frame "Core: Cleanup" {
        n116 = Unbundle By Name(w308) -> ("Core.ProcessSyncQueue"=w309:refnum<queue>, "Core.Events"=w306:T11)
        n117 = Unregister For Events(event registration refnum=w306) -> (error out=w305:errorcluster)  [unwired: 1 in]
        n118 = flat-sequence {
          tunnel: [w315] -> w307
          tunnel: w309 -> [w314]
          tunnel: w305 -> [w313]
          frame #0 {
            n119 = Enqueue Element(queue=w314, element="Finished") -> (error out=w316:errorcluster)  [unwired: 2 in, 2 out]
            n120 = Merge Errors(w316, w313) -> (w315:errorcluster)
          }
        }
      }
      frame "---------- EIS ----------" {
      }
      frame "EIS: Initialize" {
        n121 = Unbundle By Name(w324) -> ("EIS Parameters"=w323:T4)
        n122 = call "Generate Profile.vi"("error in (no error)"=w330, "EIS Parameters"=w323) -> ("error out"=w329:errorcluster, "EIS Profile"=w322:waveform(dbl)[], "Voltage Profile out"=w325:waveform(dbl)[], "Current Profile out"=w326:waveform(dbl)[], "Frequencies"=w320:dbl[])  [unwired: 5 in]
        n123 = local write "EIS Tab Control"(T1."PROFILE" ("EIS Tab Control")) -> ()
        n124 = Bundle By Name(cluster=w324, "Frequencies"=w320, "EIS Profile State"=enum16{"Idle", "Start", "Run", "Stop"}."Idle", "Voltage Profile"=w326, "Current Profile"=w325) -> (w328:T5)
        n125 = property on="EIS Profile" class="WFGraph (strict)"("Value"=w322) -> ()  [unwired: 2 in, 2 out]
      }
      frame "EIS: Start Profile" {
        n126 = local write "EIS Tab Control"(T1."RUNNING" ("EIS Tab Control")) -> ()
        n127 = Bundle By Name(cluster=w335, "EIS Profile State"=enum16{"Idle", "Start", "Run", "Stop"}."Start") -> (w334:T5)
      }
      frame "EIS: Stop Profile" {
        n128 = Bundle By Name(cluster=w340, "EIS Profile State"=enum16{"Idle", "Start", "Run", "Stop"}."Stop") -> (w339:T5)
      }
      frame "EIS: Profile Complete" {
        n129 = Unbundle By Name(w347) -> ("Profile Complete Event"=w352:refnum<user-event>, "EIS TDMS Path"=w345:path)
        n130 = Path To String(path=w345) -> (string=w344:string)
        n131 = Format Into String(format string="EIS Profile data saved to %s" ("event data"), w344) -> (resulting string=w350:string)  [unwired: 2 in, 1 out]
        n132 = Generate User Event(user event=w352, event data cluster=w350, error in=w349) -> (error out=w348:errorcluster)  [unwired: 1 in, 1 out]
        n133 = Bundle By Name(cluster=w347, "EIS Profile State"=enum16{"Idle", "Start", "Run", "Stop"}."Idle") -> (w346:T5)
      }
      frame "EIS: Generate Plots" {
        n134 = Unbundle By Name(w363) -> ("EIS TDMS Path"=w362:path, "EIS Parameters"=w354:T4)
        n135 = call "Generate EIS Plots.vi"("error in (no error)"=w361, "EIS Parameters"=w354, "TDMS Data File"=w362) -> ("error out"=w359:errorcluster, "EIS Bode Magnitude"=→"EIS Magnitude":cluster{dbl[], dbl[]}, "EIS Bode Phase"=→"EIS Phase":cluster{dbl[], dbl[]}, "EIS Nyquist"=→"EIS Nyquist":cluster{dbl[], dbl[]})  [unwired: 5 in]
        n136 = local write "EIS Tab Control"(T1."NYQUIST" ("EIS Tab Control")) -> ()
        n137 = property on="Save EIS Report" class="Bool"("DisabledEnum"=T8."Enabled" ("Disabled")) -> ()  [unwired: 2 in, 2 out]
      }
      frame "EIS: Save Report" {
        n138 = call "File Dialog"("error in"=w373, "pattern (all files)"="*.html", "pattern label"="HTML Report") -> ("selected path"=w366:path, "cancelled"=w370:bool, "error out"=w368:errorcluster)  [unwired: 9 in, 1 out]
        n139 = Or(x=w370, y=w368) -> (x .or. y?=w369:bool)
        n140 = case shown="False" w369 {
          tunnel: w368 -> [w427 w429]
          tunnel: w367 -> [w422 _]
          tunnel: w366 -> [w415 _]
          tunnel: [w409 w429] -> w365
          frame False {
            w413 = enum16{".jpg", ".png"}.".png" ("image file type (.jpg)")
            n141 = property on="Running Status Log" class="LstBox (strict)"() -> ("Item Names"=w412:string[])  [unwired: 2 in, 2 out]
            n142 = call <vilib>:"Create Report.vi"("report type"=Report_Type."HTML", "error in (no error)"=w427) -> ("report out"=w425:refnum<class "NI_report.lvclass">, "error out"=w426:errorcluster)  [unwired: 12 in]
            n143 = call-dynamic "Set Report Header Text.vi"("report in"=w425, "left header text"="HPS17K Panel", "center header text"="EIS Report", "right header text"=w422, "error in (no error)"=w426) -> ("report out"=w398:refnum<class "NI_report.lvclass">, "error out"=w399:errorcluster)  [unwired: 9 in]
            n144 = call-dynamic "Append Horizontal Line to Report.vi"("report in"=w398, "error in (no error)"=w399) -> ("report out"=w396:refnum<class "NI_report.lvclass">, "error out"=w397:errorcluster)  [unwired: 12 in]
            n145 = control-ref of="EIS Profile"() -> (w408:refnum<vi>)
            n146 = call-dynamic "Append List to Report.vi"("report in"=w396, "list elements"=w412, "error in (no error)"=w397) -> ("report out"=w394:refnum<class "NI_report.lvclass">, "error out"=w395:errorcluster)  [unwired: 9 in, 2 out]
            n147 = control-ref of="EIS Magnitude"() -> (w418:refnum<vi>)
            n148 = control-ref of="EIS Phase"() -> (w419:refnum<vi>)
            n149 = control-ref of="EIS Nyquist"() -> (w420:refnum<vi>)
            n150 = control-ref of="EIS Parameters"() -> (w400:refnum<vi>)
            n151 = call-dynamic "Append Horizontal Line to Report.vi"("report in"=w394, "error in (no error)"=w395) -> ("report out"=w392:refnum<class "NI_report.lvclass">, "error out"=w393:errorcluster)  [unwired: 12 in]
            n152 = call-dynamic "Append Control Image to Report.vi"("report in"=w392, "ctrl reference"=w400, "description"="EIS Parameters", "error in (no error)"=w393) -> ("report out"=w390:refnum<class "NI_report.lvclass">, "error out"=w391:errorcluster)  [unwired: 8 in, 2 out]
            n153 = call-dynamic "Append Horizontal Line to Report.vi"("report in"=w390, "error in (no error)"=w391) -> ("report out"=w388:refnum<class "NI_report.lvclass">, "error out"=w389:errorcluster)  [unwired: 12 in]
            n154 = call-dynamic "Append Control Image to Report.vi"("report in"=w388, "image file type (.jpg)"=w413, "ctrl reference"=w408, "description"="EIS Profile", "error in (no error)"=w389) -> ("report out"=w386:refnum<class "NI_report.lvclass">, "error out"=w387:errorcluster)  [unwired: 7 in, 2 out]
            n155 = call-dynamic "Append Horizontal Line to Report.vi"("report in"=w386, "error in (no error)"=w387) -> ("report out"=w384:refnum<class "NI_report.lvclass">, "error out"=w385:errorcluster)  [unwired: 12 in]
            n156 = call-dynamic "Append Control Image to Report.vi"("report in"=w384, "image file type (.jpg)"=w413, "ctrl reference"=w420, "description"="EIS Nyquist", "error in (no error)"=w385) -> ("report out"=w382:refnum<class "NI_report.lvclass">, "error out"=w383:errorcluster)  [unwired: 7 in, 2 out]
            n157 = call-dynamic "Append Horizontal Line to Report.vi"("report in"=w382, "error in (no error)"=w383) -> ("report out"=w380:refnum<class "NI_report.lvclass">, "error out"=w381:errorcluster)  [unwired: 12 in]
            n158 = call-dynamic "Append Control Image to Report.vi"("report in"=w380, "image file type (.jpg)"=w413, "ctrl reference"=w419, "description"="EIS Phase", "error in (no error)"=w381) -> ("report out"=w379:refnum<class "NI_report.lvclass">, "error out"=w376:errorcluster)  [unwired: 7 in, 2 out]
            n159 = call-dynamic "Append Horizontal Line to Report.vi"("report in"=w379, "error in (no error)"=w376) -> ("report out"=w378:refnum<class "NI_report.lvclass">, "error out"=w377:errorcluster)  [unwired: 12 in]
            n160 = call-dynamic "Append Control Image to Report.vi"("report in"=w378, "image file type (.jpg)"=w413, "ctrl reference"=w418, "description"="EIS Magnitude", "error in (no error)"=w377) -> ("report out"=w406:refnum<class "NI_report.lvclass">, "error out"=w407:errorcluster)  [unwired: 7 in, 2 out]
            n161 = call-dynamic "Append User Formatted HTML to Report.vi"("report in"=w406, "HTML text"="<style>body {background-color:#111111;color:#ECECED}</style>", "error in (no error)"=w407) -> ("report out"=w404:refnum<class "NI_report.lvclass">, "error out"=w405:errorcluster)  [unwired: 11 in]
            n162 = call-dynamic "Save Report to File.vi"("report in"=w404, "report file path"=w415, "prompt to replace? (F)"=TRUE, "error in (no error)"=w405) -> ("report out"=w411:refnum<class "NI_report.lvclass">, "error out"=w410:errorcluster)  [unwired: 10 in]
            n163 = call-poly <vilib>:"Open HTML Report in Browser.vi"("report in"=w411, "error in (no error)"=w410) -> ("error out"=w409:errorcluster)  [unwired: 11 in, 2 out]
          }
          frame True {
          }
        }
      }
      frame "---------- UI ----------" {
      }
      frame "UI: Front Panel State" {
        n164 = case shown="\"Close\"" w434 {
          frame "Open", Default {
            n165 = property class="VI"() -> ("FP.State"=w437:T10)  [unwired: 2 in, 2 out]
            n166 = case shown="Default" w437 {
              frame Default {
                n167 = invoke class="VI" method="FP.Open"("Activate"=TRUE, "State"=T10."Standard") -> ()  [unwired: 3 in, 5 out]
              }
              frame "Standard" {
              }
            }
          }
          frame "Close" {
            n168 = property class="VI"() -> ("FP.State"=w440:T10)  [unwired: 2 in, 2 out]
            n169 = case shown="Default" w440 {
              frame "Closed" {
              }
              frame Default {
                n170 = invoke class="VI" method="FP.Close"() -> ()  [unwired: 3 in, 3 out]
              }
            }
          }
        }
      }
      frame "UI: Initialize" {
        w442 = cluster{dbl[], dbl[]} {[], []} ("EIS Nyquist")
        n171 = property class="VI"() -> ("Name"=w457:string)  [unwired: 2 in, 2 out]
        n172 = Match Pattern(string=w457, regular expression="\\2Evi$") -> (before substring=w455:string)  [unwired: 1 in, 3 out]
        n173 = local write "EIS Tab Control"(T1."PROFILE" ("EIS Tab Control")) -> ()
        n174 = property on="Running Status Log" class="LstBox (strict)"("Item Names"=string[] []) -> ()  [unwired: 2 in, 2 out]
        n175 = Reverse String(1:w455) -> (0:w454:string)
        n176 = Match Pattern(string=w454, regular expression=":") -> (before substring=w452:string, after substring=w451:string)  [unwired: 1 in, 2 out]
        n177 = local write "EIS Profile"(waveform(dbl)[] [] ("EIS Profile")) -> ()
        n178 = local write "EIS Magnitude"(w442) -> ()
        n179 = local write "EIS Phase"(w442) -> ()
        n180 = local write "EIS Nyquist"(w442) -> ()
        n181 = Match Pattern(string=w451, regular expression="\\2E") -> (after substring=w449:string)  [unwired: 1 in, 3 out]
        n182 = Reverse String(1:w449) -> (0:w448:string)
        n183 = Reverse String(1:w452) -> (0:w447:string)
        n184 = Format Into String(format string="%s %s", w448, w447) -> (resulting string=w446:string)  [unwired: 2 in, 1 out]
        n185 = property class="VI"("Front Panel.Title"=w446) -> ()  [unwired: 2 in, 2 out]
        n186 = property on="Save EIS Report" class="Bool"("DisabledEnum"=T8."Disabled and Grayed Out" ("Disabled")) -> ()  [unwired: 2 in, 2 out]
      }
      frame "UI: Cleanup" {
        n187 = property class="VI"() -> (error out=w462:errorcluster, "FP.State"=w464:T10)  [unwired: 2 in, 1 out]
        n188 = case shown="\"Standard\", Default" w464 {
          frame "Closed" {
          }
          frame "Standard", Default {
            n189 = invoke class="VI" method="FP.Close"() -> ()  [unwired: 3 in, 3 out]
          }
        }
      }
      frame "---------- CMD ----------" {
      }
      frame "CMD: Exit" {
      }
      frame "CMD: Front Panel State" {
        n190 = Format Into String(format string="UI: Front Panel State>>%s" ("string"), w473) -> (resulting string=w472:string)  [unwired: 2 in, 1 out]
        n191 = call <vilib>:"Add State(s) to Queue__jki_lib_state_machine.vi"("State(s) in (\"\")"=w476, "State(s) at Back (\"\")"=w472) -> ("States Out"=w475:string)  [unwired: 13 in]
      }
      frame "CMD: Start Profile" {
        n192 = Unbundle By Name(w484) -> ("Profile Complete Event"=w487:refnum<user-event>, "Core.Data"=w488:variant)
        n193 = call <vilib>:"Add State(s) to Queue__jki_lib_state_machine.vi"("State(s) in Front (\"\")"="EIS: Start Profile", "State(s) in (\"\")"=w481) -> ("States Out"=w480:string)  [unwired: 13 in]
        n194 = Variant To Data(error in=w486, type=w487, Variant=w488) -> (data=w482:refnum<user-event>, error out=w485:errorcluster)
        n195 = Bundle By Name(cluster=w484, "Profile Complete Event"=w482) -> (w483:T5)
      }
      frame "CMD: Generate Plots" {
        n196 = call <vilib>:"Add State(s) to Queue__jki_lib_state_machine.vi"("State(s) in Front (\"\")"="EIS: Generate Plots", "State(s) in (\"\")"=w491) -> ("States Out"=w490:string)  [unwired: 13 in]
      }
      frame "CMD: Stop Profile" {
        n197 = call <vilib>:"Add State(s) to Queue__jki_lib_state_machine.vi"("State(s) in Front (\"\")"="EIS: Stop Profile", "State(s) in (\"\")"=w495) -> ("States Out"=w494:string)  [unwired: 13 in]
      }
    }
  }
  "error out" <- w4
  "reference out" <- "reference in"
